vi "midi_winapi_idtech1.vi"(9 "stop":bool, 10 "Beat(Hz)":i32=140) -> (0 "error out":errorcluster, 2 "MIDI output handle":i32)   [LabVIEW 2014]
uses:
  Controls/Ctrl_SysERR.ctl
  winmm.dll
panel:
  out "MIDI device number":i32
  out "midi_open_ret":T1 items=["MMSYSERR_NOERROR", "MMSYSERR_ERROR", "MMSYSERR_BADDEVICEID", "MMSYSERR_NOTENABLED", "MMSYSERR_ALLOCATED", "MMSYSERR_INVALHANDLE", "MMSYSERR_NODRIVER", "MMSYSERR_NOMEM", "MMSYSERR_NOTSUPPORTED", "MMSYSERR_BADERRNUM", "MMSYSERR_INVALFLAG", "MMSYSERR_INVALPARAM", "MMSYSERR_HANDLEBUSY", "MMSYSERR_INVALIDALIAS", "MMSYSERR_BADDB", "MMSYSERR_KEYNOTFOUND", "MMSYSERR_READERROR", "MMSYSERR_WRITEERROR", "MMSYSERR_DELETEERROR", "MMSYSERR_VALNOTFOUND", "MMSYSERR_NODRIVERCB", "MMSYSERR_MOREDATA", "MMSYSERR_LASTERROR"]
  out "Slide":i32(slide) scale=0.0..100.0
  out "Event":u8 format="%.0x"
  out "Note":u8
  out "Vol":u8
  out "Chan":u8
  out "count":i32
  out "Graph":u8[][](graph)
  in  "error in":errorcluster
  in  "Maps":enum16{"E1M1", "E1M2", "E1M3", "E1M9"}(ring)
  out "Events":i32
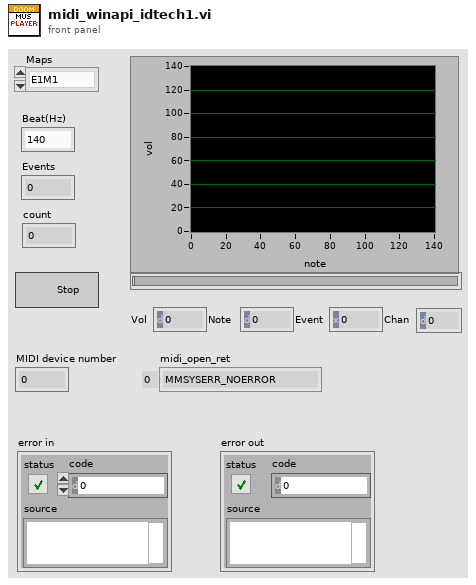
[diagram p1: front panel]
types:
  T1 = typedef "Ctrl_SysERR.ctl" = u16
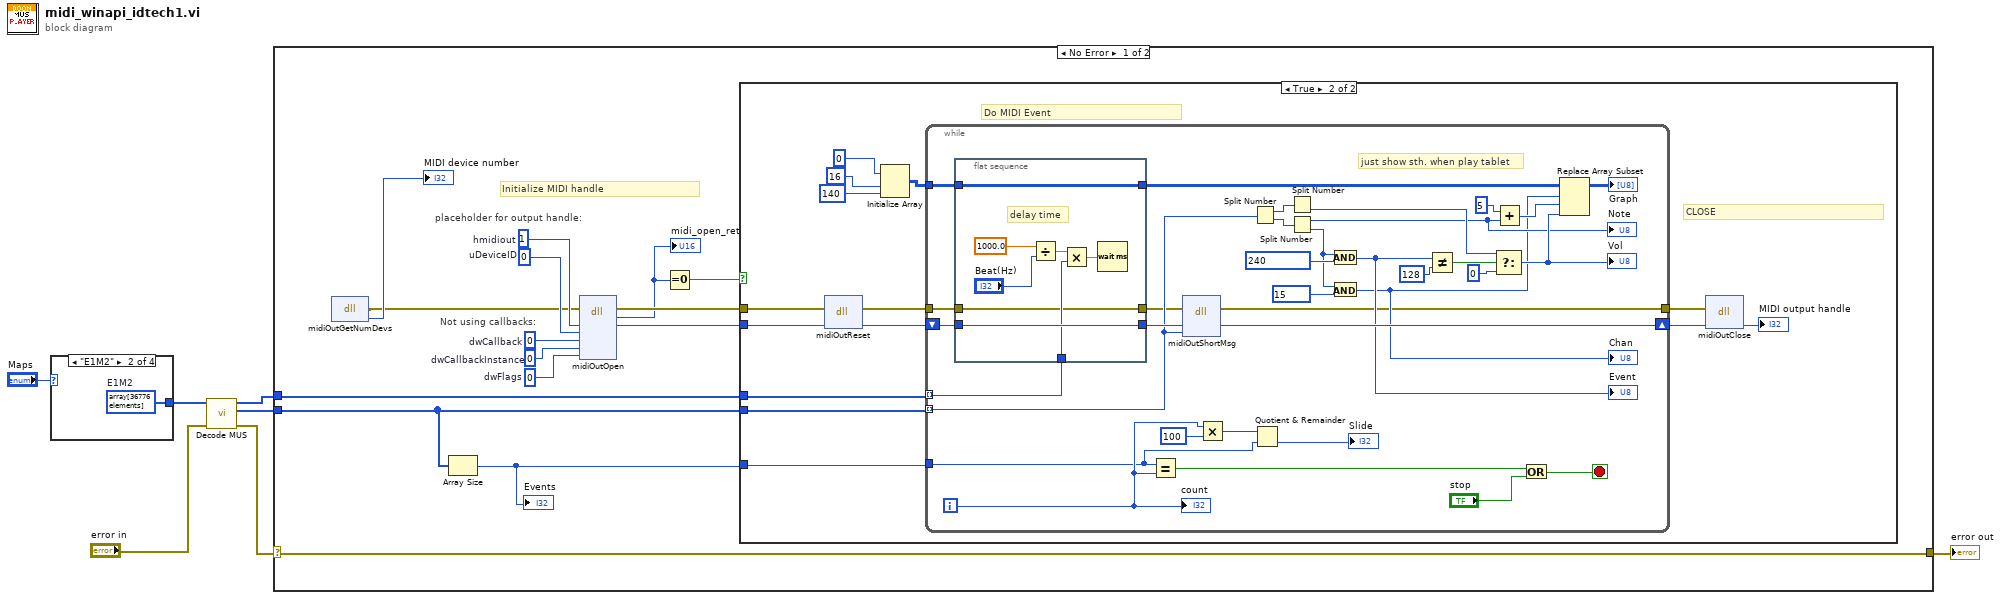
[diagram p0: block diagram]
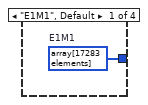
[diagram p2: hidden frame]
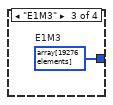
[diagram p3: hidden frame]
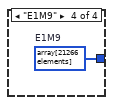
[diagram p4: hidden frame]
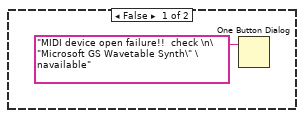
[diagram p5: hidden frame]
diagram:
  n1 = case shown="\"E1M2\"" "Maps" {
    tunnel: [w8 w9 w10 w11] -> w2
    frame "E1M1", Default {
      w8 = u8[] array[17283 elements]  # E1M1
    }
    frame "E1M2" {
      w9 = u8[] array[36776 elements]  # E1M2
    }
    frame "E1M3" {
      w10 = u8[] array[19276 elements]  # E1M3
    }
    frame "E1M9" {
      w11 = u8[] array[21266 elements]  # E1M9
    }
  }
  n2 = call "Decode MUS.vi"("error in"="error in", "Music_Lump in"=w2) -> ("error out"=w5:errorcluster, "midi_Msg"=w6:u32[], "delay"=w7:u32[])  [unwired: 7 in]
  n3 = case shown="No Error" w5 {
    selector: w5 -> [w18 w84]
    tunnel: w7 -> [w21 _]
    tunnel: w6 -> [w20 _]
    tunnel: [w18 w84] -> w4
    frame No Error {
      w25 = 0  # uDeviceID
      w22 = 0  # dwFlags
      w23 = 0  # dwCallbackInstance
      w24 = 0  # dwCallback
      w26 = 1  # hmidiout
      # "Initialize MIDI handle"
      # "placeholder for output handle:"
      # "Not using callbacks:"
      n4 = dll-call lib="winmm.dll" fn="midiOutGetNumDevs"() -> (error out=w12:errorcluster, "return type"=→"MIDI device number":i32)  [unwired: 3 in, 1 out]
      n5 = Array Size(array=w20) -> (size(s)=w19:i32)
      "Events" <- w19
      n6 = dll-call lib="winmm.dll" fn="midiOutOpen"(error in=w12, "hmidiout"=w26, "uDeviceID"=w25, "dwCallback"=w24, "dwCallbackInstance"=w23, "dwFlags"=w22) -> (error out=w17:errorcluster, w14:i32, "hmidiout"=w16:i32)  [unwired: 6 in, 1 out]
      "midi_open_ret" <- w14
      n7 = Equal To 0?(x=w14) -> (x = 0?=w13:bool)
      n8 = case shown="True" w13 {
        tunnel: w21 -> [_ w39]
        tunnel: w20 -> [_ w38]
        tunnel: w19 -> [_ w37]
        tunnel: w17 -> [_ w32]
        tunnel: w16 -> [_ w29]
        frame False {
          n9 = One Button Dialog(message="MIDI device open failure!!  check \n\"Microsoft GS Wavetable Synth\" \navailable") -> ()  [unwired: 1 in, 1 out]
        }
        frame True {
          # "Do MIDI Event"
          # "CLOSE"
          n10 = dll-call lib="winmm.dll" fn="midiOutReset"(error in=w32, "hmidiout"=w29) -> (error out=w31:errorcluster, "hmidiout"=w28:i32)  [unwired: 3 in, 1 out]
          n11 = Initialize Array(u8 0, 16 ("index"), 140 ("index")) -> (w33:u8[][])
          n12 = while {
            shift-right: [w75] -> w40
            shift-left: w28 -> [w74]
            tunnel: w39 -> [w71] mode=indexing
            tunnel: w38 -> [w67] mode=indexing
            tunnel: w37 -> [w45]
            tunnel: w33 -> [w68]
            tunnel: w31 -> [w43]
            tunnel: [w42] -> w30
            i -> [w46]
            stop <- w72 stop-if-true
            # "just show sth. when play tablet"
            n13 = flat-sequence {
              tunnel: w74 -> [w83]
              tunnel: [w83] -> w73
              tunnel: w71 -> [w78]
              tunnel: w68 -> [w77]
              tunnel: [w77] -> w59
              tunnel: [w76] -> w44
              tunnel: w43 -> [w76]
              frame #0 {
                # "delay time"
                n14 = Divide(x=1000.0, y="Beat(Hz)") -> (x/y=w82:dbl)
                n15 = Multiply(x=w82, y=w78) -> (x*y=w79:dbl)
                n16 = Wait (ms)(milliseconds to wait=w79) -> ()  [unwired: 1 out]
              }
            }
            n17 = Equal?(x=w45, y=w46) -> (x = y?=w70:bool)
            n18 = dll-call lib="winmm.dll" fn="midiOutShortMsg"(error in=w44, "hmidiout"=w73, "data"=w67) -> (error out=w42:errorcluster, "hmidiout"=w75:i32)  [unwired: 4 in, 1 out]
            n19 = Multiply(x=w46, y=100) -> (x*y=w48:i32)
            n20 = Split Number(x=w67) -> (hi(x)=w66:u16, lo(x)=w65:u16)
            n21 = Quotient & Remainder(x=w48, y=w45) -> (floor(x/y)=→"Slide":i32)  [unwired: 1 out]
            n22 = Split Number(x=w66) -> (lo(x)=w58:u8)  [unwired: 1 out]
            n23 = Split Number(x=w65) -> (hi(x)=w51:u8, lo(x)=w62:u8)
            "Note" <- w51
            n24 = And(x=w62, y=u8 240 ("f")) -> (x .and. y?=w52:u8)
            "Event" <- w52
            n25 = And(x=w62, y=u8 15 ("f")) -> (x .and. y?=w50:u8)
            "Chan" <- w50
            n26 = Not Equal?(x=w52, y=u8 128) -> (x != y?=w61:bool)
            n27 = Select(t=w58, s=w61, f=u8 0) -> (s? t:f=w57:u8)
            "Vol" <- w57
            n28 = Add(x=u8 5, y=w51) -> (x+y=w55:u8)
            n29 = Or(x=w70, y="stop") -> (x .or. y?=w72:bool)
            n30 = Replace Array Subset(array=w59, new element=w57, index (row)=w50, index (col)=w55) -> (→"Graph":u8[][])
            "count" <- w46
          }
          n31 = dll-call lib="winmm.dll" fn="midiOutClose"(error in=w30, "hmidiout"=w40) -> ("hmidiout"=→"MIDI output handle":i32)  [unwired: 3 in, 2 out]
        }
      }
    }
    frame Error {
    }
  }
  "error out" <- w4
